vi "Insert Start Message.vi"(8 "error in (no error)":errorcluster, 10 "Start Time":timestamp, 11 "TimeStamper in":refnum<class "TimeStamper.lvclass">) -> (0 "error out":errorcluster, 3 "TimeStamper out":refnum<class "TimeStamper.lvclass">)   [LabVIEW 2014, in "TimeStamper.lvclass"]
uses:
  TimeStamper.lvclass
  Database/SessionPrimary.ctl
  TimeStamper.lvclass/TimeStamper.ctl
  AcquistionObject/AcquistionObject.lvclass
  <vilib>/addons/database/NI_Database_API.lvlib
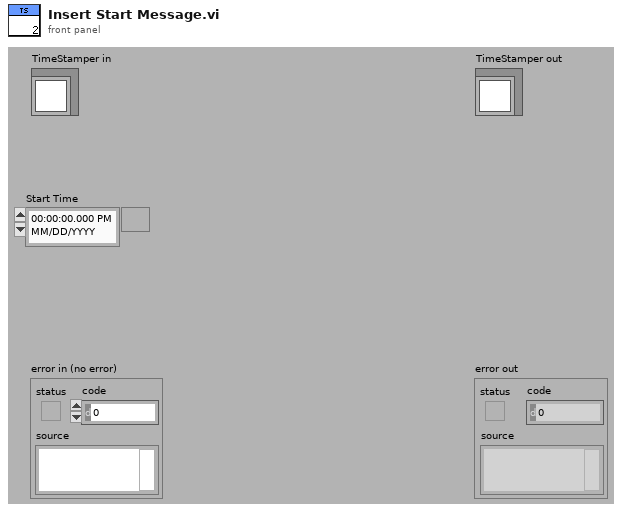
[diagram p1: front panel]
types:
  T1 = typedef "SessionPrimary.ctl" = cluster{"setup":u8, "subject_id":i32, "session_start_time":dbl}
  T2 = cluster{"setup":u8, "subject_id":i32, "experimenter":string, "session_start_time":dbl, "session_path":path, "session_datetime":timestamp, "session_stop_time":dbl}
  T3 = typedef "NI_Database_API.lvlib/Conn ObjectReference.ctl" = refnum<k1>
  T4 = cluster{"connection reference out":T3, "table":string, "columns":string[], i32}
  T5 = cluster{cluster{"connection reference out":T3, "table":string, "columns":string[], i32}, "Variant":variant}
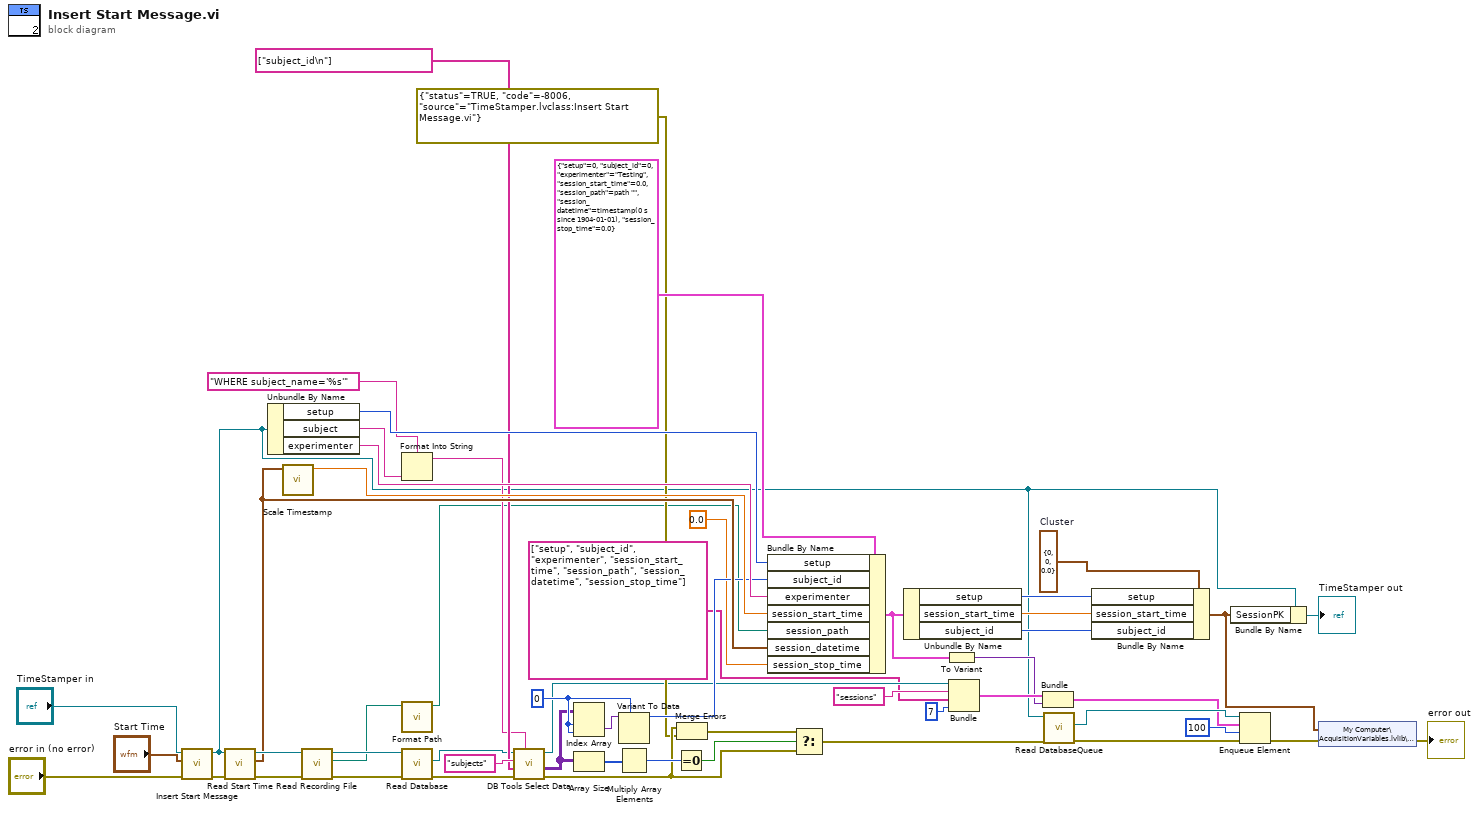
[diagram p0: block diagram]
diagram:
  w29 = 0
  w51 = T1 {"setup"=0, "subject_id"=0, "session_start_time"=0.0}  # Cluster
  n1 = call-parent "Insert Start Message.vi"("error in (no error)"="error in (no error)", "Start Time"="Start Time", "AcquistionObject in"="TimeStamper in") -> ("error out"=w46:errorcluster, "AcquistionObject out"=w6:refnum<class "TimeStamper.lvclass">)  [unwired: 7 in]
  n2 = call-dynamic "Read Start Time.vi"("error in (no error)"=w46, "AcquistionObject in"=w6) -> ("error out"=w45:errorcluster, "Start Time"=w36:timestamp, "AcquistionObject out"=w40:refnum<class "TimeStamper.lvclass">)  [unwired: 7 in]
  n3 = Unbundle By Name(w6) -> ("setup"=w48:u8, "subject"=w32:string, "experimenter"=w47:string)
  n4 = call "Scale Timestamp.vi"("Time Stamp"=w36) -> ("Scaled timestamp"=w37:dbl)  [unwired: 10 in]
  n5 = call-dynamic "Read Recording File.vi"("error in (no error)"=w45, "AcquistionObject in"=w40) -> ("error out"=w44:errorcluster, "Recording File"=w17:path, "AcquistionObject out"=w39:refnum<class "TimeStamper.lvclass">)  [unwired: 7 in]
  n6 = Format Into String(format string="WHERE subject_name='%s'", w32) -> (resulting string=w31:string)  [unwired: 2 in, 1 out]
  n7 = call "Format Path.vi"("Input path"=w17) -> ("Output path"=w16:path)  [unwired: 10 in]
  n8 = call-dynamic "Read Database.vi"("error in (no error)"=w44, "AcquistionObject in"=w39) -> ("error out"=w21:errorcluster, "reference"=w22:T3)  [unwired: 7 in, 1 out]
  n9 = call <vilib>:"DB Tools Select Data.vi"("condition"=w31, "error in (no error)"=w21, "columns"=string[] ["subject_id\n"], "table"="subjects", "connection reference"=w22) -> ("error out"=w20:errorcluster, "data"=w27:variant[][], "connection reference out"=w13:T3)  [unwired: 1 in]
  n10 = Index Array(array=w27, index (row)=w29, index (col)=w29) -> (element=w30:variant)
  n11 = Array Size(array=w27) -> (size(s)=w26:i32[])
  n12 = Variant To Data(type=w29, Variant=w30) -> (data=w28:i32)  [unwired: 1 in, 1 out]
  n13 = Multiply Array Elements(1:w26) -> (0:w25:i32)
  n14 = Equal To 0?(x=w25) -> (x = 0?=w24:bool)
  n15 = Merge Errors(w20, errorcluster {"status"=TRUE, "code"=-8006, "source"="TimeStamper.lvclass:Insert Start Message.vi"} ("error in")) -> (w23:errorcluster)
  n16 = Bundle By Name(cluster=T2 {"setup"=0, "subject_id"=0, "experimenter"="Testing", "session_start_time"=0.0, "session_path"=path "", "session_datetime"=timestamp(0 s since 1904-01-01), "session_stop_time"=0.0} ("Cluster"), "setup"=w48, "subject_id"=w28, "experimenter"=w47, "session_start_time"=w37, "session_path"=w16, "session_datetime"=w36, "session_stop_time"=0.0) -> (w10:T2)
  n17 = Select(t=w23, s=w24, f=w20) -> (s? t:f=w2:errorcluster)
  n18 = Unbundle By Name(w10) -> ("setup"=w50:u8, "session_start_time"=w49:dbl, "subject_id"=w18:i32)
  n19 = To Variant(anything=w10) -> (Variant=w9:variant)
  n20 = Bundle("connection reference out"=w13, "table"="sessions", "columns"=string[] ["setup", "subject_id", "experimenter", "session_start_time", "session_path", "session_datetime", "session_stop_time"], 7) -> (w14:T4)  [unwired: 1 in]
  n21 = Bundle(w14, "Variant"=w9) -> (w5:T5)  [unwired: 1 in]
  n22 = call-dynamic "Read DatabaseQueue.vi"("error in (no error)"=w2, "AcquistionObject in"=w6) -> ("error out"=w8:errorcluster, "DatabaseQueue"=w7:refnum<queue>)  [unwired: 7 in, 1 out]
  n23 = Bundle By Name(cluster=w51, "setup"=w50, "session_start_time"=w49, "subject_id"=w18) -> (w43:T1)
  n24 = Bundle By Name(cluster=w6, "SessionPK"=w43) -> (→"TimeStamper out":refnum<class "TimeStamper.lvclass">)
  n25 = Enqueue Element(queue=w7, element=w5, timeout in ms (-1)=100, error in (no error)=w8) -> (error out=w3:errorcluster)  [unwired: 2 out]
  n26 = shared-variable "My Computer\\AcquisitionVariables.lvlib\\SessionPK"(w43, error in=w3) -> (error out=→"error out":errorcluster)
